vi "Logitech_DA_JoyStick_Map.vi"(0 "JoystickDevRef":T3) -> (1 "AxesCluster":T2, 2 "ButtonsCluster":T1)   [LabVIEW 2014]
uses:
  <vilib>/Rock Robotics/WPI/Joystick/WPI_JoystickDevRef.ctl
  <vilib>/Rock Robotics/WPI/Joystick/WPI_JoystickDeviceEnum.ctl
  <vilib>/Rock Robotics/Network Tables/SD Write Numeric Array.vi
  <vilib>/Rock Robotics/Network Tables/SD Write Boolean Array.vi
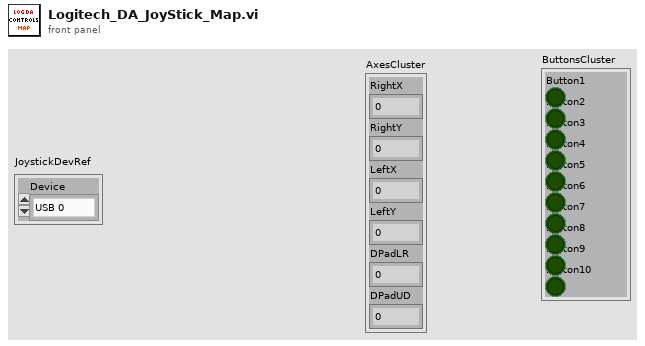
[diagram p1: front panel]
types:
  T1 = cluster{"Button1":bool, "Button2":bool, "Button3":bool, "Button4":bool, "Button5":bool, "Button6":bool, "Button7":bool, "Button8":bool, "Button9":bool, "Button10":bool}
  T2 = cluster{"RightX":dbl, "RightY":dbl, "LeftX":dbl, "LeftY":dbl, "DPadLR":dbl, "DPadUD":dbl}
  T3 = typedef "WPI_JoystickDevRef.ctl" = cluster{"Device":T4}
  T4 = typedef "WPI_JoystickDeviceEnum.ctl" = enum16{"USB 0", "USB 1", "USB 2", "USB 3", "USB 4", "USB 5"}
  T5 = cluster{"upper limit":dbl, "upper limit":dbl, "upper limit":dbl, "upper limit":dbl, "upper limit":dbl, "upper limit":dbl}
  T6 = cluster{bool, bool, bool, bool, bool, bool, bool, bool, bool, bool}
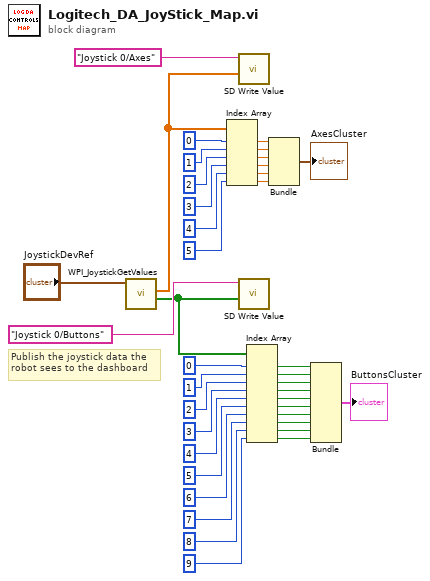
[diagram p0: block diagram]
diagram:
  # "Publish the joystick data the\nrobot sees to the dashboard"
  n1 = call <vilib>:"WPI_JoystickGetValues.vi"("JoystickDevRef"="JoystickDevRef") -> ("Buttons"=w33:bool[], "Axes"=w38:dbl[])  [unwired: 6 in, 3 out]
  n2 = Index Array(array=w38, index #1=0, index #2=1, index #3=2 ("index"), index #4=3 ("index"), index #5=4 ("index"), index #6=5 ("index")) -> (element #1=w20:dbl, element #2=w19:dbl, element #3=w18:dbl, element #4=w17:dbl, element #5=w14:dbl, element #6=w13:dbl)
  n3 = call-poly <vilib>:"SD Write Value.vi"("Numeric Array"=w38, "Name"="Joystick 0/Axes") -> ()  [unwired: 8 in, 2 out]
  n4 = call-poly <vilib>:"SD Write Value.vi"("Boolean Array"=w33, "Name"="Joystick 0/Buttons") -> ()  [unwired: 8 in, 2 out]
  n5 = Index Array(array=w33, index #1=0, index #2=1, index #3=2 ("index"), index #4=3 ("index"), index #5=4 ("index"), index #6=5 ("index"), index #7=6 ("index"), index #8=7 ("index"), index #9=8 ("index"), index #10=9 ("index")) -> (element #1=w11:bool, element #2=w10:bool, element #3=w9:bool, element #4=w8:bool, element #5=w7:bool, element #6=w6:bool, element #7=w5:bool, element #8=w4:bool, element #9=w3:bool, element #10=w2:bool)
  n6 = Bundle("upper limit"=w20, "upper limit"=w19, "upper limit"=w18, "upper limit"=w17, "upper limit"=w14, "upper limit"=w13) -> (→"AxesCluster":T5)  [unwired: 1 in]
  n7 = Bundle(w11, w10, w9, w8, w7, w6, w5, w4, w3, w2) -> (→"ButtonsCluster":T6)  [unwired: 1 in]
